vi "SWERVE EXEC CRNR.vi"(0 "swerve STEER motors":T1[](array[typedef]) {"gear ratio" format="%_5f"; "MOTOR SELECT" items=["REV NEO"=5676, "REV NEO 550"=11000, "VEX Falcon"=6380, "WC Kraken"=6000]}, 1 "Swerve refs":T19(array[cluster]), 2 "Swerve position":T18(ring), 5 "swerve DRIVE motors":T7[](array[typedef]) {"gear ratio" format="%_5f"; "MOTOR SELECT" items=["REV NEO"=5676, "REV NEO 550"=11000, "VEX Falcon"=6380, "WC Kraken"=6000]}, 9 "speed norm":dbl[](array[numeric]), 12 "angle":dbl[](array[numeric]), 14 "swerve module data":T10[](array[typedef]) {"corner wt (lbm)" format="%_4f"; "POS" format="%.3g"; "coord wrt geom CTR"."Y" format="%.4g"; "coord wrt geom CTR"."X" format="%.4g"; "from pivot to module"."theta park (deg)" format="%.4g"; "from pivot to module"."theta spin (deg)" format="%.4g"; "from pivot to module"."theta (deg)" format="%.4g"; "from pivot to module"."R" format="%.4g"; "ABS" format="%.3g"; "target" format="%.3g"; "V" format="%.3g"}) -> (4 "swerve module out":T10 {"corner wt (lbm)" format="%_4f"; "POS" format="%.3g"; "coord wrt geom CTR"."Y" format="%.4g"; "coord wrt geom CTR"."X" format="%.4g"; "from pivot to module"."theta park (deg)" format="%.4g"; "from pivot to module"."theta spin (deg)" format="%.4g"; "from pivot to module"."theta (deg)" format="%.4g"; "from pivot to module"."R" format="%.4g"; "ABS" format="%.3g"; "target" format="%.3g"; "V" format="%.3g"}, 6 "velocity out":dbl, 8 "steer angle out\n(deg)":dbl)   [LabVIEW 2023]
uses:
  <vilib>/Rock Robotics/WPI/ThirdParty/Phoenix-LabVIEW/Motor Controller/Controls/CTRE_Phoenix_MotorControl_ControlMode.ctl
  ctrl defs/ctrl MOTOR SELECT.ctl
  <vilib>/Rock Robotics/WPI/ThirdParty/Phoenix-LabVIEW/Motor Controller/Controls/CTRE_Phoenix_MotorControl_TalonFXInvertType.ctl
  <vilib>/Rock Robotics/WPI/ThirdParty/Phoenix-LabVIEW/Motor Controller/Controls/CTRE_Phoenix_MotorControl_NeutralMode.ctl
  <vilib>/Rock Robotics/WPI/ThirdParty/REV Robotics/REVLib/Typedef/Spark MAX Smart Motion Parameters.ctl
  ctrl defs/ctrl motor PIDF coefficients.ctl
  ctrl defs/ctrl Talon FX config.ctl
  ctrl defs/ctrl Spark MAX current limiting.ctl
  <vilib>/Rock Robotics/WPI/ThirdParty/REV Robotics/REVLib/Typedef/Spark MAX Idle Mode.ctl
  ctrl defs/ctrl swerve motor.ctl
  ctrl defs/ctrl swerve module.ctl
  <vilib>/Rock Robotics/SystemInterfaces/DIO/FPGA_DIOPWMChannel.ctl
  <vilib>/Rock Robotics/WPI/PWM/WPI_PWMDeadband.ctl
  <vilib>/Rock Robotics/WPI/MotorControl/WPI_MotorControlType.ctl
  <vilib>/Rock Robotics/SystemInterfaces/DIO/FPGA_DIOChannel.ctl
  <vilib>/Rock Robotics/WPI/MotorControl/WPI_MotorControlDeviceRef.ctl
  <vilib>/Rock Robotics/WPI/ThirdParty/Phoenix-LabVIEW/CANCoder/Controls/CTRE_Phoenix_CANcoder_DeviceRef.ctl
panel:
  in  "swerve mod\ndata":T17 {"swerve STEER motor"."gear ratio" format="%_5f"; "swerve STEER motor"."MOTOR SELECT" items=["REV NEO"=5676, "REV NEO 550"=11000, "VEX Falcon"=6380, "WC Kraken"=6000]; "swerve DRIVE motor"."gear ratio" format="%_5f"; "swerve DRIVE motor"."MOTOR SELECT" items=["REV NEO"=5676, "REV NEO 550"=11000, "VEX Falcon"=6380, "WC Kraken"=6000]; "swerve module"."corner wt (lbm)" format="%_4f"; "swerve module"."POS" format="%.3g"; "swerve module"."coord wrt geom CTR"."Y" format="%.4g"; "swerve module"."coord wrt geom CTR"."X" format="%.4g"; "swerve module"."from pivot to module"."theta park (deg)" format="%.4g"; "swerve module"."from pivot to module"."theta spin (deg)" format="%.4g"; "swerve module"."from pivot to module"."theta (deg)" format="%.4g"; "swerve module"."from pivot to module"."R" format="%.4g"; "swerve module"."ABS" format="%.3g"; "swerve module"."target" format="%.3g"; "swerve module"."V" format="%.3g"}
  out "error out":errorcluster
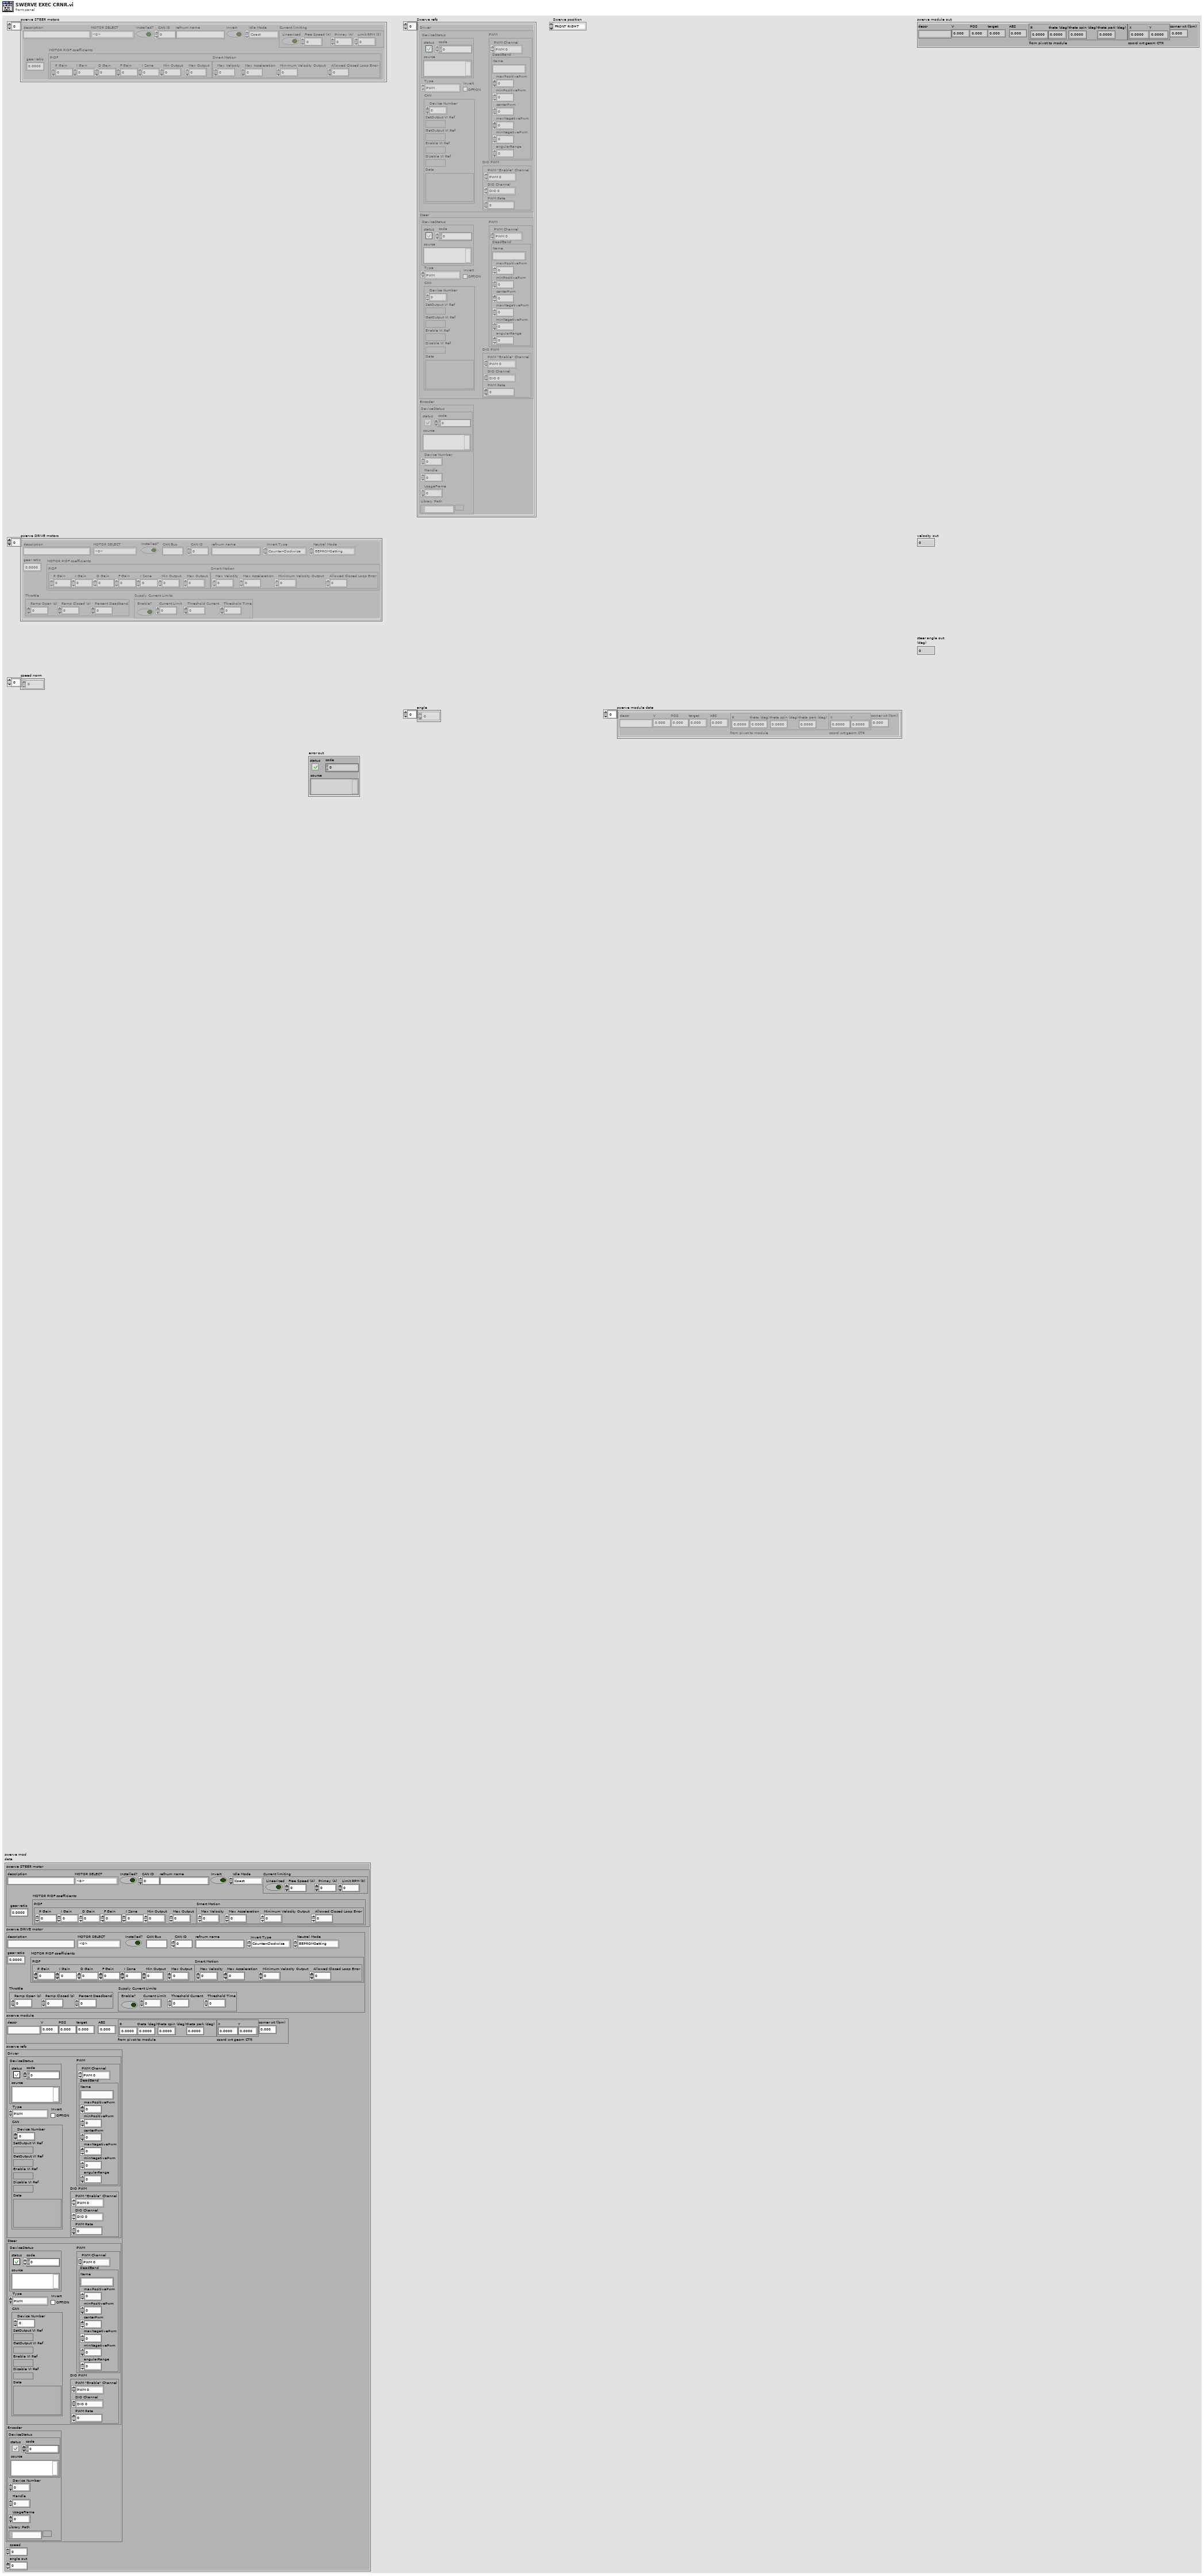
[diagram p1: front panel]
types:
  T1 = typedef "ctrl swerve motor.ctl" = cluster{"description":string, "MOTOR SELECT":T2, "Installed?":bool, "CAN ID":u8, "refnum name":string, "Invert":bool, "Idle Mode":T3, "Current limiting":T4, "MOTOR PIDF coefficients":T5, "gear ratio":dbl}
  T2 = typedef "ctrl MOTOR SELECT.ctl" = i16
  T3 = typedef "Spark MAX Idle Mode.ctl" = enum16{"Coast", "Brake"}
  T4 = typedef "ctrl Spark MAX current limiting.ctl" = cluster{"Linearized":bool, "Free Speed (A)":dbl, "Primay (A)":dbl, "Limit RPM (0)":u32}
  T5 = typedef "ctrl motor PIDF coefficients.ctl" = cluster{"PIDF":cluster{"P Gain":dbl, "I Gain":dbl, "D Gain":dbl, "F Gain":dbl, "I Zone":dbl, "Min Output":dbl, "Max Output":dbl}, "Smart Motion":T6}
  T6 = typedef "Spark MAX Smart Motion Parameters.ctl" = cluster{"Max Velocity":dbl, "Max Acceleration":dbl, "Minimum Velocity Output":dbl, "Allowed Closed Loop Error":dbl}
  T7 = typedef "ctrl Talon FX config.ctl" = cluster{"refnum name":string, "CAN ID":u8, "Installed?":bool, "description":string, "MOTOR SELECT":T2, "CAN Bus":string, "Invert Type":T8, "Neutral Mode":T9, "gear ratio":dbl, "MOTOR PIDF coefficients":T5, "Throttle":cluster{"Ramp Open (s)":dbl, "Ramp Closed (s)":dbl, "Percent Deadband":dbl}, "Supply Current Limits":cluster{"Enable?":bool, "Current Limit":dbl, "Threshold Current":dbl, "Threshold Time":dbl}}
  T8 = typedef "CTRE_Phoenix_MotorControl_TalonFXInvertType.ctl" = enum16{"Counter-Clockwise", "Clockwise"}
  T9 = typedef "CTRE_Phoenix_MotorControl_NeutralMode.ctl" = enum8{"EEPROMSetting", "Override to Coast", "Override to Brake"}
  T10 = typedef "ctrl swerve module.ctl" = cluster{"descr":string, "V":dbl, "POS":dbl, "target":dbl, "ABS":dbl, "from pivot to module":cluster{"R":dbl, "theta (deg)":dbl, "theta spin (deg)":dbl, "theta park (deg)":dbl}, "coord wrt geom CTR":cluster{"X":dbl, "Y":dbl}, "corner wt (lbm)":dbl}
  T11 = typedef "WPI_MotorControlDeviceRef.ctl" = cluster{"DeviceStatus":errorcluster, "Type":T12, "PWM":cluster{"PWM Channel":T13, "DeadBand":T14}, "CAN":cluster{"Device Number":u8, "SetOutput VI Ref":variant, "GetOutput VI Ref":variant, "Enable VI Ref":variant, "Disable VI Ref":variant, "Data":variant}, "Invert":bool, "DIO PWM":cluster{"PWM \"Enable\" Channel":T13, "DIOChannel":T15, "PWM Rate":dbl}}
  T12 = typedef "WPI_MotorControlType.ctl" = enum16{"PWM", "CAN", "DIO PWM"}
  T13 = typedef "FPGA_DIOPWMChannel.ctl" = enum8{"PWM 0", "PWM 1", "PWM 2", "PWM 3", "PWM 4", "PWM 5", "PWM 6", "PWM 7", "PWM 8", "PWM 9", "PWM MXP 0", "PWM MXP 1", "PWM MXP 2", "PWM MXP 3", "PWM MXP 4", "PWM MXP 5", "PWM MXP 6", "PWM MXP 7", "PWM MXP 8", "PWM MXP 9", "Invalid"}
  T14 = typedef "WPI_PWMDeadband.ctl" = cluster{"Name":string, "maxPositivePwm":i32, "minPositivePwm":i32, "centerPwm":i32, "maxNegativePwm":i32, "minNegativePwm":i32, "angularRange":u16}
  T15 = typedef "FPGA_DIOChannel.ctl" = enum8{"DIO 0", "DIO 1", "DIO 2", "DIO 3", "DIO 4", "DIO 5", "DIO 6", "DIO 7", "DIO 8", "DIO 9", "DIO MXP 0", "DIO MXP 1", "DIO MXP 2", "DIO MXP 3", "DIO MXP 4", "DIO MXP 5", "DIO MXP 6", "DIO MXP 7", "DIO MXP 8", "DIO MXP 9", "DIO MXP 10", "DIO MXP 11", "DIO MXP 12", "DIO MXP 13", "DIO MXP 14", "DIO MXP 15", "SPI Port CS1", "SPI Port CS2", "SPI Port CS3", "SPI Port MISO", "SPI Port MOSI", "Invalid"}
  T16 = typedef "CTRE_Phoenix_CANcoder_DeviceRef.ctl" = cluster{"DeviceStatus":errorcluster, "Device Number":u8, "Handle":u64, "UsageFrame":u32, "Library Path":path}
  T17 = cluster{"swerve STEER motor":T1, "swerve DRIVE motor":T7, "swerve module":T10, "swerve refs":cluster{"Driver":T11, "Steer":T11, "Encoder":T16}, "speed":dbl, "angle out":dbl}
  T18 = enum16{"FRONT RIGHT", "FRONT LEFT", "REAR LEFT", "REAR RIGHT"}
  T19 = cluster{"Driver":T11, "Steer":T11, "Encoder":T16}[]
  T20 = cluster{"Driver":T11, "Steer":T11, "Encoder":T16}
  T21 = typedef "CTRE_Phoenix_MotorControl_ControlMode.ctl" = u16
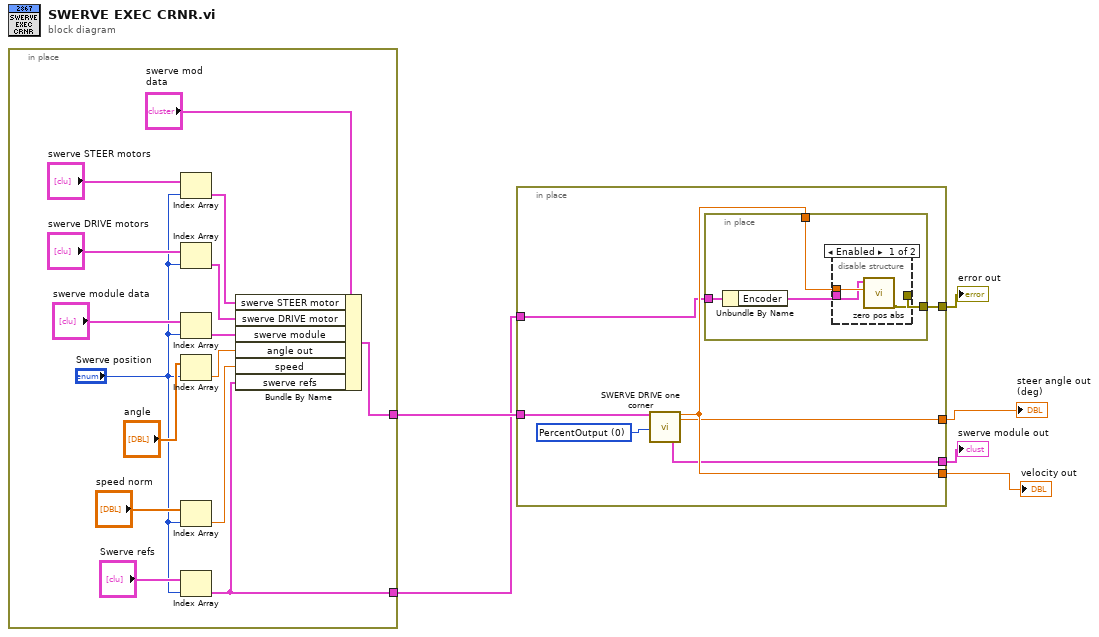
[diagram p0: block diagram]
diagram:
  n1 = in-place {
    in-place-border: [w8] -> w4
    in-place-border: [w7] -> w3
    n2 = Index Array(array="swerve STEER motors", index="Swerve position") -> (element=w20:T1)
    n3 = Index Array(array="swerve DRIVE motors", index="Swerve position") -> (element=w19:T7)
    n4 = Index Array(array="swerve module data", index="Swerve position") -> (element=w18:T10)
    n5 = Index Array(array="angle", index="Swerve position") -> (element=w17:dbl)
    n6 = Index Array(array="speed norm", index="Swerve position") -> (element=w16:dbl)
    n7 = Index Array(array="Swerve refs", index="Swerve position") -> (element=w7:T20)
    n8 = Bundle By Name(cluster="swerve mod\ndata", "swerve STEER motor"=w20, "swerve DRIVE motor"=w19, "swerve module"=w18, "angle out"=w17, "speed"=w16, "swerve refs"=w7) -> (w8:T17)
  }
  n9 = in-place {
    in-place-border: [w28] -> w2
    in-place-border: [w27] -> w1
    in-place-border: [w26] -> w5
    in-place-border: [w25] -> w6
    in-place-border: w4 -> [w23]
    in-place-border: w3 -> [w22]
    w24 = T21 0 items=["PercentOutput"=0, "Position"=1, "Velocity"=2, "Current"=3, "Follower"=5, "MotionProfile"=6, "MotionMagic"=7, "MotionProfileArc"=10, "Disabled"=15] ("Control Mode")
    n10 = call "SWERVE DRIVE one corner.vi"("swerve mod\ndata"=w23, "Control Mode"=w24) -> ("swerve module out"=w26:T10, "velocity out"=w28:dbl, "steer angle out\n(deg)"=w27:dbl)  [unwired: 14 in, 1 out]
    n11 = in-place {
      in-place-border: w28 -> [w32]
      in-place-border: w22 -> [w31]
      in-place-border: [w29] -> w25
      n12 = Unbundle By Name(w31) -> ("Encoder"=w30:T16)
      n13 = disable-structure shown="Enabled" {
        disable-tunnel: w32 -> [w35 _]
        disable-tunnel: w30 -> [w34 _]
        disable-tunnel: [w33 _] -> w29
        frame Enabled {
          n14 = call "zero pos abs.vi"("velocity"=w35, "Encoder"=w34) -> ("error out"=w33:errorcluster)  [unwired: 9 in]
        }
        frame Disabled {
        }
      }
    }
  }
  "error out" <- w6
  "swerve module out" <- w5
  "steer angle out\n(deg)" <- w1
  "velocity out" <- w2
